vi "Pcre2GetMark8.vi"(8 "error in":errorcluster, 11 "pMatchData":u64 format="%.0x") -> (0 "error out":errorcluster, 2 "Mark":string, 3 "pMatchData":u64 format="%.0x")   [LabVIEW 2021, in "libpcre2-8.lvlib"]
uses:
  libpcre2-8.lvlib
  Pcre2ErrorNull.vi
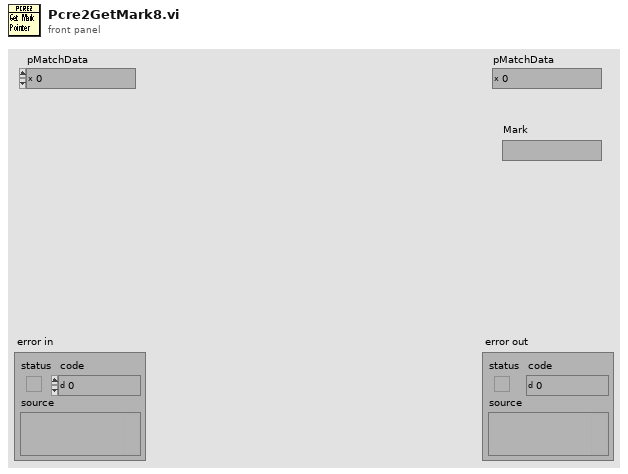
[diagram p1: front panel]
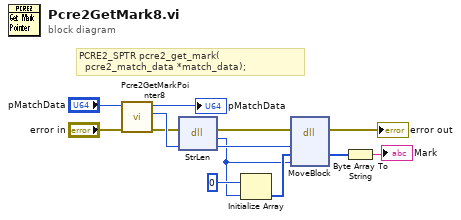
[diagram p0: block diagram]
diagram:
  # "PCRE2_SPTR pcre2_get_mark(\n  pcre2_match_data *match_data);"
  n1 = call "Pcre2GetMarkPointer8.vi"("error in"="error in", "pMatchData"="pMatchData") -> ("error out"=w6:errorcluster, "pMark"=w10:u64, "pMatchData"=→"pMatchData":u64)  [unwired: 7 in]
  n2 = dll-call lib="LabVIEW" fn="StrLen"(error in=w6, "s"=w10) -> (error out=w7:errorcluster, "size"=w1:i32, "s"=w9:u64)  [unwired: 2 in, 1 out]
  n3 = Initialize Array(u8 0 ("U8"), w1) -> (w2:u8[])
  n4 = dll-call lib="LabVIEW" fn="MoveBlock"(error in=w7, "pointerSrc"=w9, "pointerDest"=w2, "size"=w1) -> (error out=→"error out":errorcluster, "pointerDest"=w4:u8[])  [unwired: 5 in, 1 out]
  n5 = Byte Array To String(unsigned byte array=w4) -> (string=→"Mark":string)
